vi "IO.vi"() -> ()   [LabVIEW 2015]
uses:
  <userlib>/ADLINK/APS168.lvlib
panel:
  out "Tab Control":enum32{"Page 1", "Page 2", "Page 3", "Page 4"}(tab)
  out "DIO_In_0":T1
  out "DIO_In_1":T1
  out "DIO_In_2":T1
  out "DIO_In_3":T1
  out "DIO_In_4":T1
  out "DIO_In_5":T1
  out "DIO_In_6":T1
  out "DIO_In_7":T1
  in  "DIO_Out_4":T1
  in  "DIO_Out_3":T1
  in  "DIO_Out_2":T1
  in  "DIO_Out_1":T1
  in  "DIO_Out_0":T1
  in  "DIO_Out_8":T1
  in  "DIO_Out_7":T1
  in  "DIO_Out_5":T1
  in  "DIO_Out_6":T1
  in  "Radio Buttons":enum32{"上一頁", "下一頁"}(radio)
  in  "Exit":bool
  # "I/O 狀態"
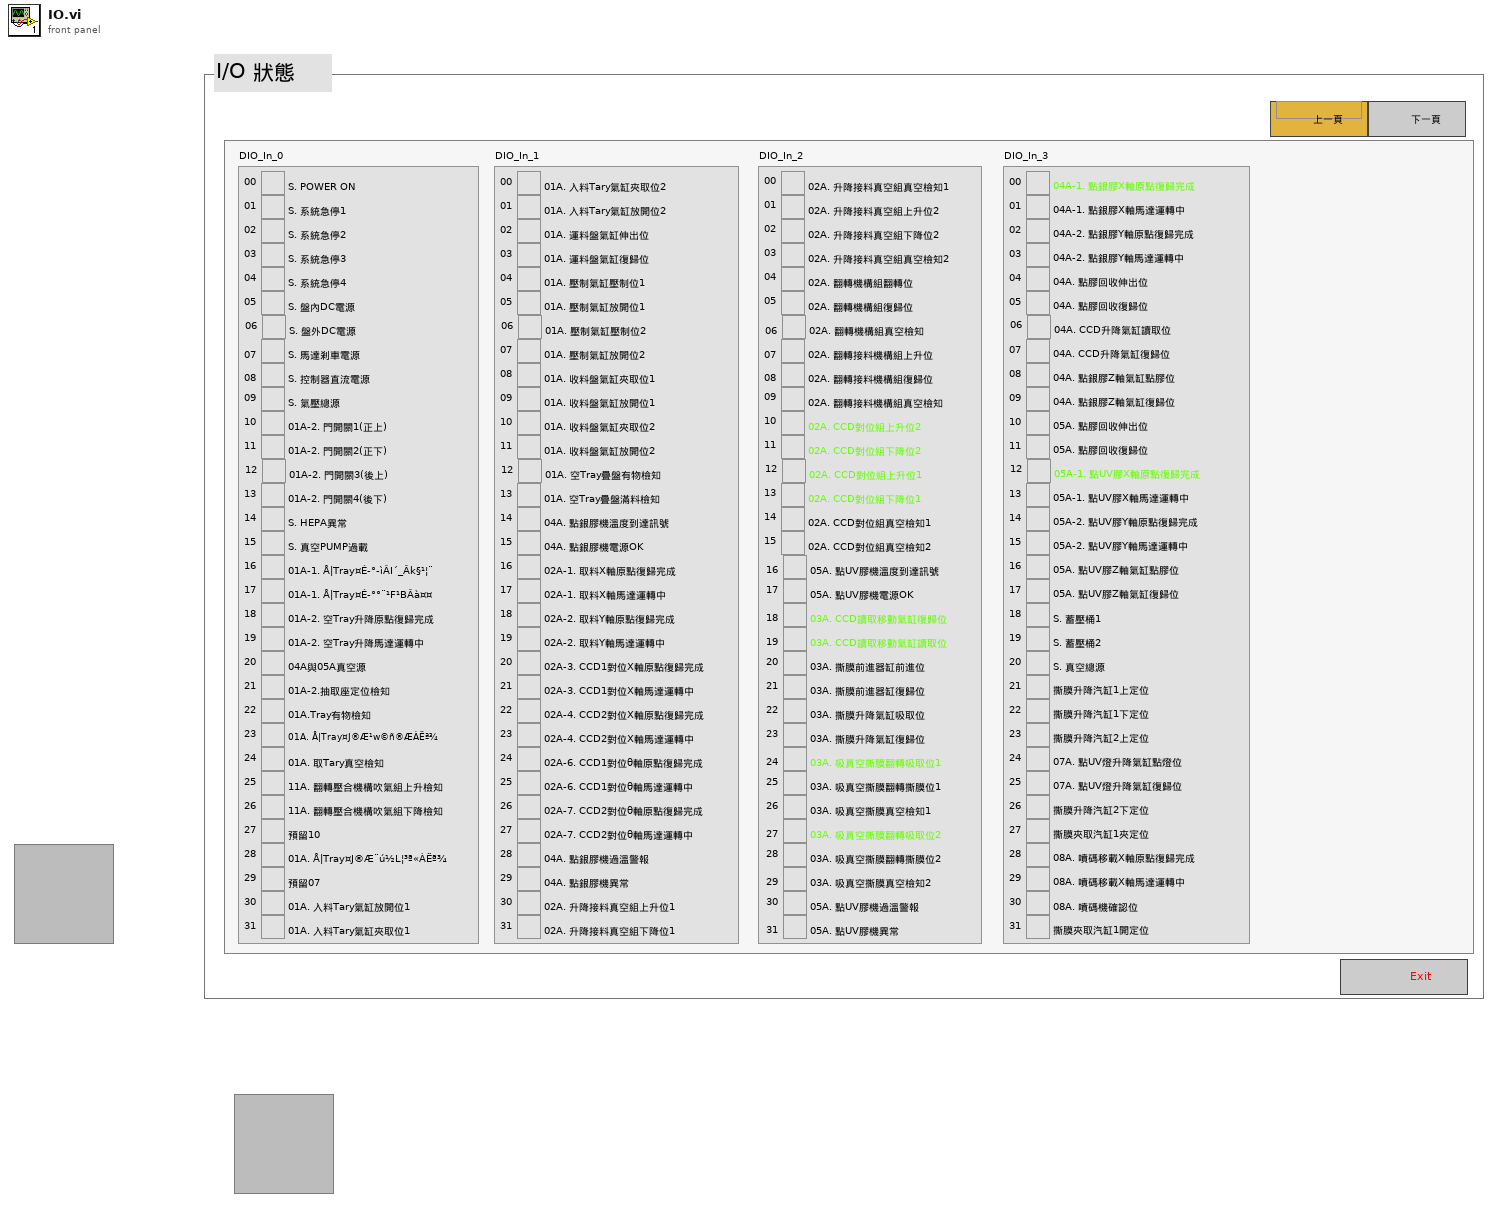
[diagram p1: front panel]
types:
  T1 = cluster{"Boolean 1":bool, "Boolean 2":bool, "Boolean 3":bool, "Boolean 4":bool, "Boolean 5":bool, "Boolean 6":bool, "Boolean 7":bool, "Boolean 8":bool, "Boolean 9":bool, "Boolean 10":bool, "Boolean 11":bool, "Boolean 12":bool, "Boolean 13":bool, "Boolean 14":bool, "Boolean 15":bool, "Boolean 16":bool, "Boolean 17":bool, "Boolean 18":bool, "Boolean 19":bool, "Boolean 20":bool, "Boolean 21":bool, "Boolean 22":bool, "Boolean 23":bool, "Boolean 24":bool, "Boolean 25":bool, "Boolean 26":bool, "Boolean 27":bool, "Boolean 28":bool, "Boolean 29":bool, "Boolean 30":bool, "30":bool, "Boolean 32":bool}
  T2 = cluster{"Boolean array[0]":bool, "Boolean array[1]":bool, "Boolean array[2]":bool, "Boolean array[3]":bool, "Boolean array[4]":bool, "Boolean array[5]":bool, "Boolean array[6]":bool, "Boolean array[7]":bool, "Boolean array[8]":bool, "Boolean array[9]":bool, "Boolean array[10]":bool, "Boolean array[11]":bool, "Boolean array[12]":bool, "Boolean array[13]":bool, "Boolean array[14]":bool, "Boolean array[15]":bool, "Boolean array[16]":bool, "Boolean array[17]":bool, "Boolean array[18]":bool, "Boolean array[19]":bool, "Boolean array[20]":bool, "Boolean array[21]":bool, "Boolean array[22]":bool, "Boolean array[23]":bool, "Boolean array[24]":bool, "Boolean array[25]":bool, "Boolean array[26]":bool, "Boolean array[27]":bool, "Boolean array[28]":bool, "Boolean array[29]":bool, "Boolean array[30]":bool, "Boolean array[31]":bool}
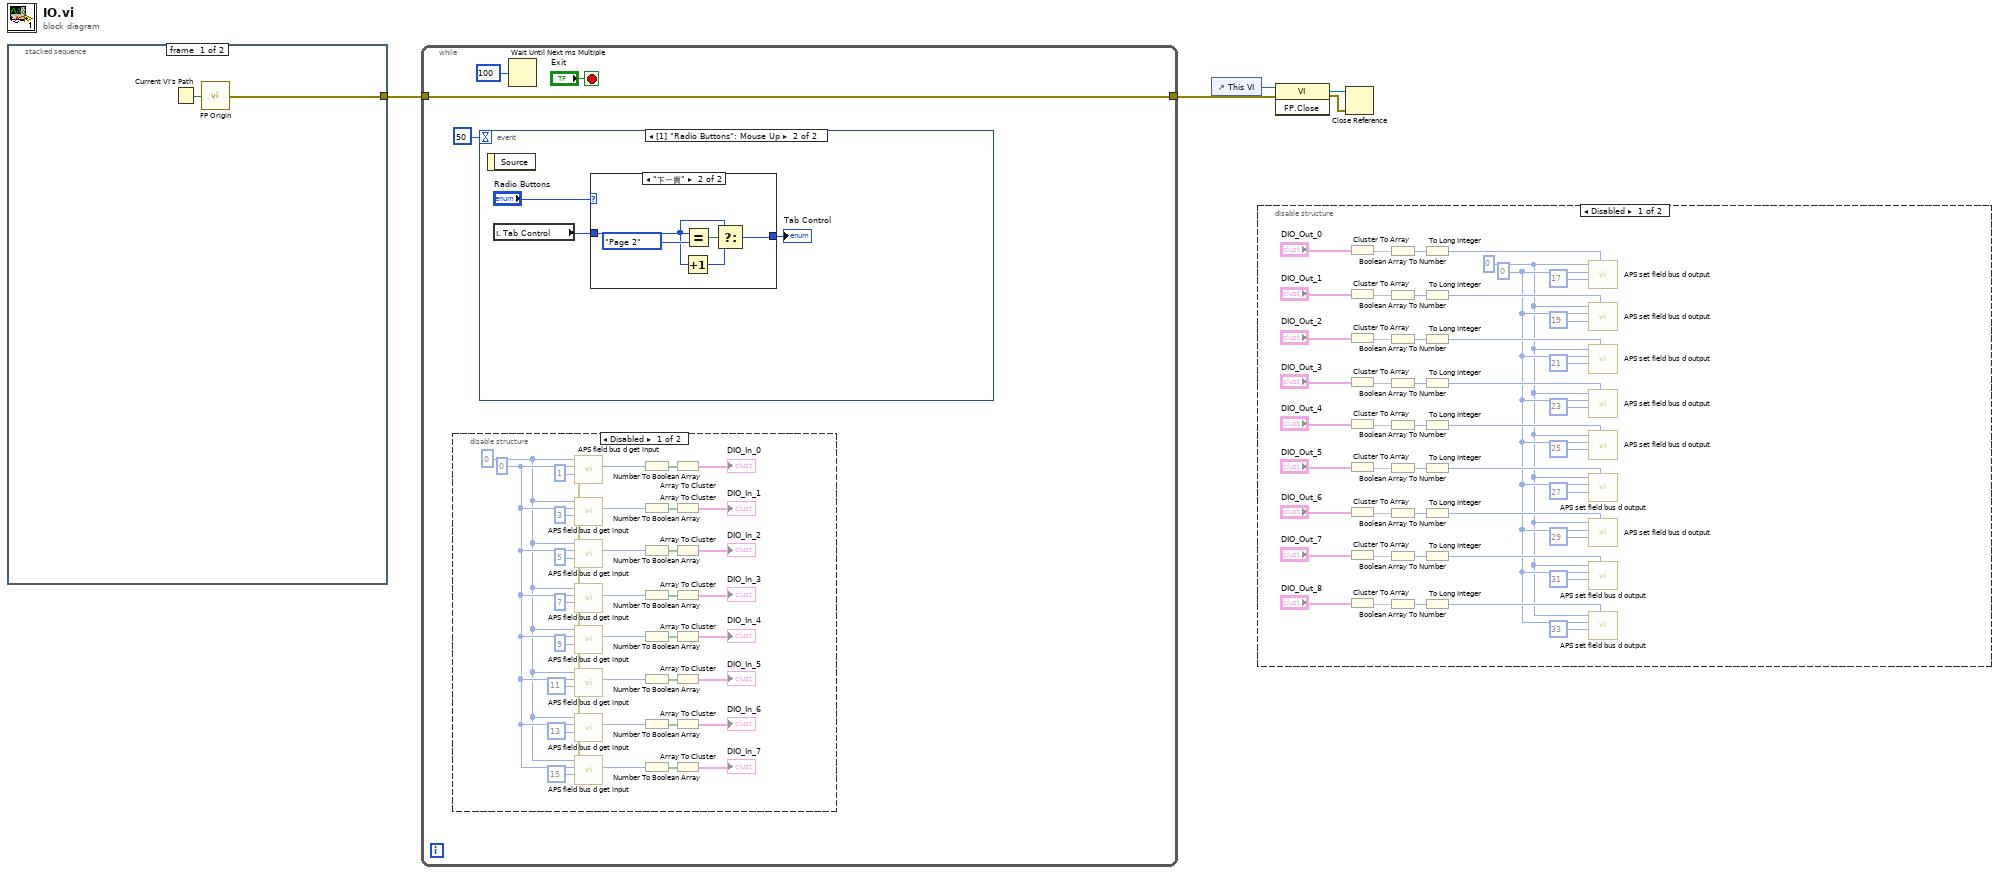
[diagram p0: block diagram]
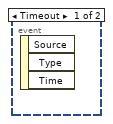
[diagram p5: hidden frame]
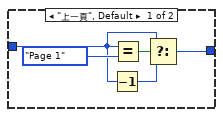
[diagram p6: hidden frame]
diagram:
  n1 = stacked-sequence {
    tunnel: [w6 _] -> w1
    frame #0 {
      n2 = Current VI's Path() -> (path=w7:path)
      n3 = call "FP Origin.vi"("vi path"=w7) -> ("error out"=w6:errorcluster)
    }
    frame #1 {
    }
  }
  n4 = while {
    tunnel: w1 -> [w9]
    tunnel: [w9] -> w5
    stop <- "Exit" stop-if-true
    n5 = disable-structure shown="Disabled" {
      frame Disabled {
        w52 = 0 ("BUS_No")
        w51 = 0 ("Board_ID")
        n6 = call <userlib>:"APS field bus d get input.vi"("MOD_No"=1, "BUS_No"=w52, "Board_ID"=w51) -> ("error out"=w44:errorcluster, "DI_Value out"=w20:i32)  [unwired: 6 in, 1 out]
        n7 = call <userlib>:"APS field bus d get input.vi"("error in (no error)"=w44, "MOD_No"=3, "BUS_No"=w52, "Board_ID"=w51) -> ("error out"=w45:errorcluster, "DI_Value out"=w16:i32)  [unwired: 5 in, 1 out]
        n8 = call <userlib>:"APS field bus d get input.vi"("error in (no error)"=w45, "MOD_No"=5, "BUS_No"=w52, "Board_ID"=w51) -> ("error out"=w46:errorcluster, "DI_Value out"=w13:i32)  [unwired: 5 in, 1 out]
        n9 = call <userlib>:"APS field bus d get input.vi"("error in (no error)"=w46, "MOD_No"=7, "BUS_No"=w52, "Board_ID"=w51) -> ("error out"=w47:errorcluster, "DI_Value out"=w23:i32)  [unwired: 5 in, 1 out]
        n10 = call <userlib>:"APS field bus d get input.vi"("error in (no error)"=w47, "MOD_No"=9, "BUS_No"=w52, "Board_ID"=w51) -> ("error out"=w48:errorcluster, "DI_Value out"=w26:i32)  [unwired: 5 in, 1 out]
        n11 = call <userlib>:"APS field bus d get input.vi"("error in (no error)"=w48, "MOD_No"=11, "BUS_No"=w52, "Board_ID"=w51) -> ("error out"=w49:errorcluster, "DI_Value out"=w29:i32)  [unwired: 5 in, 1 out]
        n12 = call <userlib>:"APS field bus d get input.vi"("error in (no error)"=w49, "MOD_No"=13, "BUS_No"=w52, "Board_ID"=w51) -> ("error out"=w50:errorcluster, "DI_Value out"=w35:i32)  [unwired: 5 in, 1 out]
        n13 = call <userlib>:"APS field bus d get input.vi"("error in (no error)"=w50, "MOD_No"=15, "BUS_No"=w52, "Board_ID"=w51) -> ("DI_Value out"=w32:i32)  [unwired: 5 in, 2 out]
        n14 = Number To Boolean Array(number=w20) -> (Boolean array=w19:bool[])
        n15 = Number To Boolean Array(number=w16) -> (Boolean array=w17:bool[])
        n16 = Number To Boolean Array(number=w13) -> (Boolean array=w12:bool[])
        n17 = Number To Boolean Array(number=w23) -> (Boolean array=w24:bool[])
        n18 = Number To Boolean Array(number=w26) -> (Boolean array=w25:bool[])
        n19 = Number To Boolean Array(number=w29) -> (Boolean array=w30:bool[])
        n20 = Number To Boolean Array(number=w35) -> (Boolean array=w36:bool[])
        n21 = Number To Boolean Array(number=w32) -> (Boolean array=w31:bool[])
        n22 = Array To Cluster(array=w19) -> (cluster=→"DIO_In_0":T2)
        n23 = Array To Cluster(array=w17) -> (cluster=→"DIO_In_1":T2)
        n24 = Array To Cluster(array=w12) -> (cluster=→"DIO_In_2":T2)
        n25 = Array To Cluster(array=w24) -> (cluster=→"DIO_In_3":T2)
        n26 = Array To Cluster(array=w25) -> (cluster=→"DIO_In_4":T2)
        n27 = Array To Cluster(array=w30) -> (cluster=→"DIO_In_5":T2)
        n28 = Array To Cluster(array=w36) -> (cluster=→"DIO_In_6":T2)
        n29 = Array To Cluster(array=w31) -> (cluster=→"DIO_In_7":T2)
      }
      frame Enabled {
      }
    }
    n30 = event shown="[1] \"Radio Buttons\": Mouse Up" {
      selector: _ -> [_ _]
      dyn-events: _ -> [_ _]
      timeout: 50 -> [_ _]
      event Timeout {
        n31 = event-data() -> ()  [unwired: 1 in, 3 out]
      }
      event "Radio Buttons": Mouse Up {
        n32 = event-data() -> ()  [unwired: 1 in, 1 out]
        n33 = local read "Tab Control"() -> (w54:enum32{"Page 1", "Page 2", "Page 3", "Page 4"})
        n34 = case shown="\"下一頁\"" "Radio Buttons" {
          tunnel: w54 -> [w56 w61]
          tunnel: [w57 w62] -> w53
          frame "上一頁", Default {
            n35 = Decrement(x=w56) -> (x-1=w58:enum32{"Page 1", "Page 2", "Page 3", "Page 4"})
            n36 = Equal?(x=w56, y=enum32{"Page 1", "Page 2", "Page 3", "Page 4"}."Page 1") -> (x = y?=w60:bool)
            n37 = Select(t=w56, s=w60, f=w58) -> (s? t:f=w57:enum32{"Page 1", "Page 2", "Page 3", "Page 4"})
          }
          frame "下一頁" {
            n38 = Increment(x=w61) -> (x+1=w63:enum32{"Page 1", "Page 2", "Page 3", "Page 4"})
            n39 = Equal?(x=w61, y=enum32{"Page 1", "Page 2", "Page 3", "Page 4"}."Page 2") -> (x = y?=w65:bool)
            n40 = Select(t=w61, s=w65, f=w63) -> (s? t:f=w62:enum32{"Page 1", "Page 2", "Page 3", "Page 4"})
          }
        }
        "Tab Control" <- w53
      }
    }
    n41 = Wait Until Next ms Multiple(millisecond multiple=u32 100) -> ()  [unwired: 1 out]
  }
  n42 = control-ref of="This VI"() -> (w4:refnum<vi>)
  n43 = disable-structure shown="Disabled" {
    frame Disabled {
      w69 = 0 ("BUS_No")
      w68 = 0 ("Board_ID")
      n44 = Cluster To Array(cluster="DIO_Out_0") -> (array=w67:bool[])
      n45 = Cluster To Array(cluster="DIO_Out_1") -> (array=w74:bool[])
      n46 = Cluster To Array(cluster="DIO_Out_2") -> (array=w85:bool[])
      n47 = Cluster To Array(cluster="DIO_Out_3") -> (array=w88:bool[])
      n48 = Cluster To Array(cluster="DIO_Out_4") -> (array=w89:bool[])
      n49 = Cluster To Array(cluster="DIO_Out_5") -> (array=w92:bool[])
      n50 = Cluster To Array(cluster="DIO_Out_6") -> (array=w93:bool[])
      n51 = Cluster To Array(cluster="DIO_Out_7") -> (array=w96:bool[])
      n52 = Cluster To Array(cluster="DIO_Out_8") -> (array=w97:bool[])
      n53 = Boolean Array To Number(Boolean array=w67) -> (number=w71:u32)
      n54 = Boolean Array To Number(Boolean array=w74) -> (number=w73:u32)
      n55 = Boolean Array To Number(Boolean array=w85) -> (number=w86:u32)
      n56 = Boolean Array To Number(Boolean array=w88) -> (number=w87:u32)
      n57 = Boolean Array To Number(Boolean array=w89) -> (number=w90:u32)
      n58 = Boolean Array To Number(Boolean array=w92) -> (number=w91:u32)
      n59 = Boolean Array To Number(Boolean array=w93) -> (number=w94:u32)
      n60 = Boolean Array To Number(Boolean array=w96) -> (number=w95:u32)
      n61 = Boolean Array To Number(Boolean array=w97) -> (number=w98:u32)
      n62 = To Long Integer(number=w71) -> (32bit integer=w72:i32)
      n63 = To Long Integer(number=w73) -> (32bit integer=w83:i32)
      n64 = To Long Integer(number=w86) -> (32bit integer=w112:i32)
      n65 = To Long Integer(number=w87) -> (32bit integer=w111:i32)
      n66 = To Long Integer(number=w90) -> (32bit integer=w110:i32)
      n67 = To Long Integer(number=w91) -> (32bit integer=w109:i32)
      n68 = To Long Integer(number=w94) -> (32bit integer=w108:i32)
      n69 = To Long Integer(number=w95) -> (32bit integer=w107:i32)
      n70 = To Long Integer(number=w98) -> (32bit integer=w106:i32)
      n71 = call <userlib>:"APS set field bus d output.vi"("DO_Value"=w72, "MOD_No"=17, "BUS_No"=w69, "Board_ID"=w68) -> ()  [unwired: 6 in, 2 out]
      n72 = call <userlib>:"APS set field bus d output.vi"("DO_Value"=w83, "MOD_No"=19, "BUS_No"=w69, "Board_ID"=w68) -> ()  [unwired: 6 in, 2 out]
      n73 = call <userlib>:"APS set field bus d output.vi"("DO_Value"=w112, "MOD_No"=21, "BUS_No"=w69, "Board_ID"=w68) -> ()  [unwired: 6 in, 2 out]
      n74 = call <userlib>:"APS set field bus d output.vi"("DO_Value"=w111, "MOD_No"=23, "BUS_No"=w69, "Board_ID"=w68) -> ()  [unwired: 6 in, 2 out]
      n75 = call <userlib>:"APS set field bus d output.vi"("DO_Value"=w110, "MOD_No"=25, "BUS_No"=w69, "Board_ID"=w68) -> ()  [unwired: 6 in, 2 out]
      n76 = call <userlib>:"APS set field bus d output.vi"("DO_Value"=w109, "MOD_No"=27, "BUS_No"=w69, "Board_ID"=w68) -> ()  [unwired: 6 in, 2 out]
      n77 = call <userlib>:"APS set field bus d output.vi"("DO_Value"=w108, "MOD_No"=29, "BUS_No"=w69, "Board_ID"=w68) -> ()  [unwired: 6 in, 2 out]
      n78 = call <userlib>:"APS set field bus d output.vi"("DO_Value"=w107, "MOD_No"=31, "BUS_No"=w69, "Board_ID"=w68) -> ()  [unwired: 6 in, 2 out]
      n79 = call <userlib>:"APS set field bus d output.vi"("DO_Value"=w106, "MOD_No"=33, "BUS_No"=w69, "Board_ID"=w68) -> ()  [unwired: 6 in, 2 out]
    }
    frame Enabled {
    }
  }
  n80 = invoke class="VI" method="FP.Close"(reference=w4, error in=w5) -> (reference out=w3:refnum<vi>, error out=w2:errorcluster)  [unwired: 1 in, 1 out]
  n81 = Close Reference(reference=w3, error in (no error)=w2) -> ()  [unwired: 1 out]
